vi "ChannelPropertiesHierarchy(numeric).vi"(11 "ChannelName":string) -> (3 "PropertiesHierarchy(numeric)":string[][](array[string]))   [LabVIEW 2013, in "TektronixDPO.lvclass"]
doc: "Return the properties hierarcy for the specified channel (only for numeric type properties)"
uses:
  TektronixDPO.lvclass
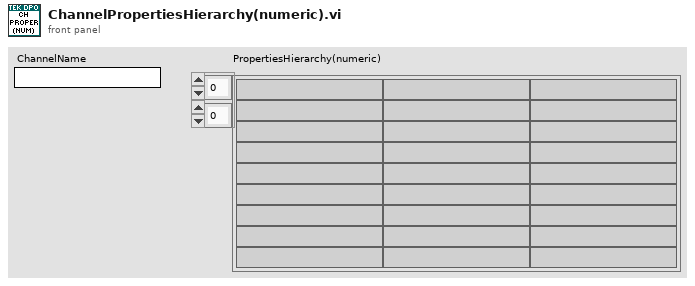
[diagram p1: front panel]
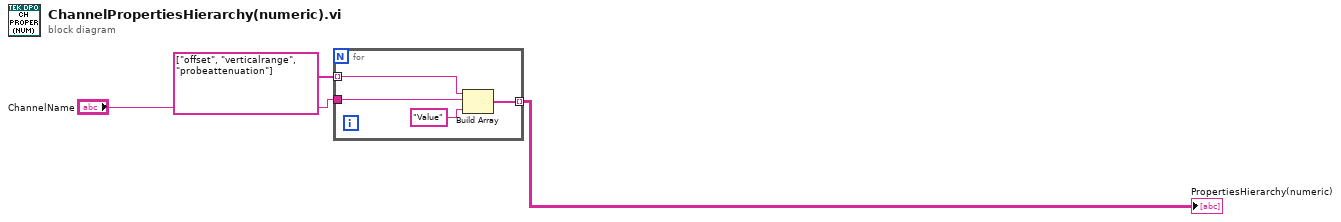
[diagram p0: block diagram]
diagram:
  n1 = for {
    tunnel: [w7] -> w3 mode=indexing
    tunnel: "ChannelName" -> [w5]
    tunnel: string[] ["offset", "verticalrange", "probeattenuation"] -> [w4] mode=indexing
    n2 = Build Array(w4, w5, "Value" ("Element Name")) -> (w7:string[])
  }
  "PropertiesHierarchy(numeric)" <- w3
